vi "testErr.vi"(8 "error in (no error)":errorcluster, 9 "OutputString":string) -> (0 "error out":errorcluster, 1 "TestStr":string)   [LabVIEW 2020]
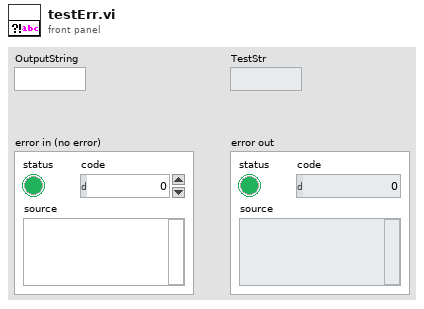
[diagram p1: front panel]
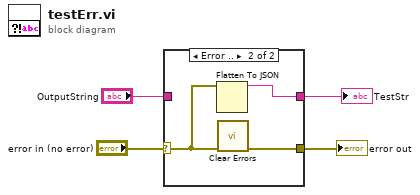
[diagram p0: block diagram]
diagram:
  n1 = case shown="Error .." "error in (no error)" {
    selector: "error in (no error)" -> [w5 w8]
    tunnel: "OutputString" -> [w6 _]
    tunnel: [w6 w7] -> w2
    tunnel: [w5 w9] -> w1
    frame No Error {
    }
    frame Error {
      n2 = Flatten To JSON(anything=w8) -> (JSON string=w7:string)  [unwired: 2 in, 1 out]
      n3 = call <vilib>:"Clear Errors.vi"("error in (no error)"=w8) -> ("error out"=w9:errorcluster)  [unwired: 5 in, 1 out]
    }
  }
  "error out" <- w1
  "TestStr" <- w2
